vi "Untitled 5.vi"() -> ()   [LabVIEW 2018]
panel:
  out "hi(x)":u8 format="%.0x"
  out "lo(x)":u8 format="%.0x"
  out "string":string
  in  "dado":u16=4 format="%.0x"
  in  "opcode":u8=4
  in  "addr":u8=4
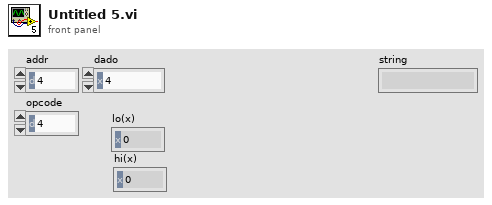
[diagram p1: front panel]
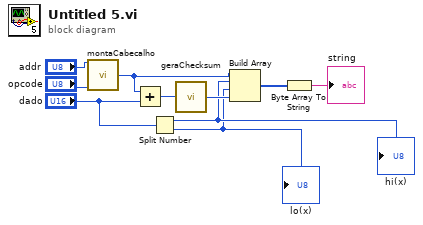
[diagram p0: block diagram]
diagram:
  n1 = call "montaCabecalho.vi"("addr"="addr", "opcode"="opcode") -> ("Cabeçalho"=w2:u8)  [unwired: 13 in]
  n2 = Add(x=w2, y="dado") -> (x+y=w8:u16)
  n3 = Split Number(x="dado") -> (hi(x)=w6:u8, lo(x)=w5:u8)
  "lo(x)" <- w5
  "hi(x)" <- w6
  n4 = call "geraChecksum.vi"("Soma"=w8) -> ("checksum"=w10:u8)  [unwired: 14 in]
  n5 = Build Array(w2, w6, w5, w10) -> (w9:u8[])
  n6 = Byte Array To String(unsigned byte array=w9) -> (string=→"string":string)
